vi "Maui 2.0.GetSubpanels.vi"(6 "timeout in ms (-1)":i32, 8 "error in (no error)":errorcluster, 11 "Maui 2.0":refnum<class "Maui 2.0.lvclass">) -> (0 "error out":errorcluster, 2 "Subpanels":refnum<class "SMO.lvclass">[](array[class]), 3 "Maui 2.0 out":refnum<class "Maui 2.0.lvclass">)   [LabVIEW 2020, in "Maui 2.0.lvclass"]
doc: "---------------------------------------------------------------\nJKI State Machine Objects™\nhttp://jki.net/state-machine-objects/\nCopyright (C) 2005-2015, JKI <info@jki.net>\nALL RIGHTS RESERVEDJKI State Machine Objects (SMO) 1.0.0.4\nJKI - JKI\nCopyright (c) 2015, JKI"
uses:
  Maui 2.0.lvclass
  C:/Program Files (x86)/National Instruments/LabVIEW 2020/vi.lib/JKI/JKI SMO/SMO/SMO.lvclass
  <vilib>/JKI/JKI SMO/SMO/SMO.lvclass
  Maui 2.0.lvclass/Maui 2.0.ctl
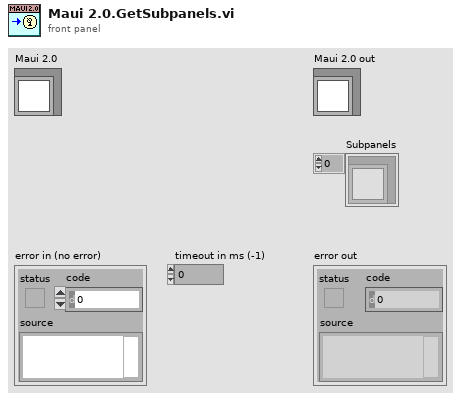
[diagram p1: front panel]
types:
  T1 = typedef "SMO.lvclass/SMOState --Enum.ctl" = enum16{"unknown", "Created", "Started", "Stopped"}
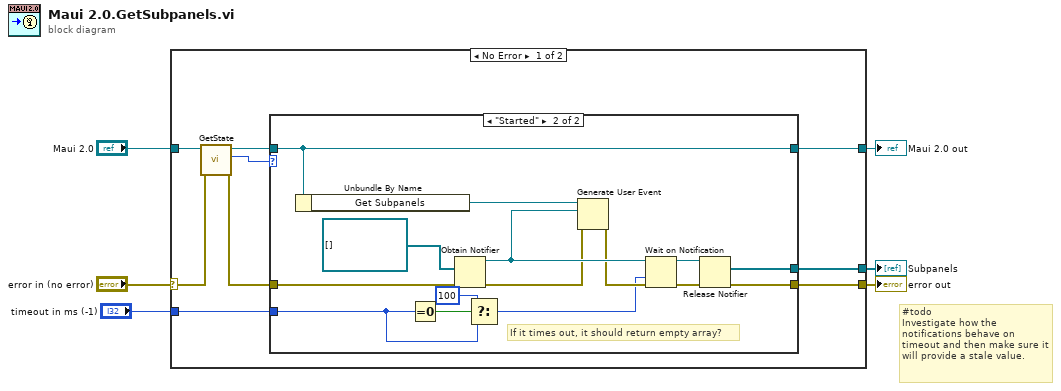
[diagram p0: block diagram]
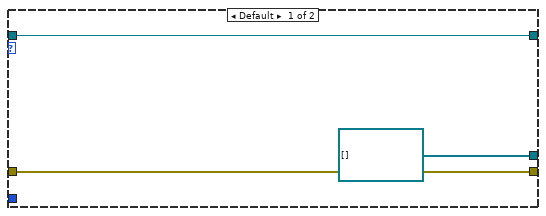
[diagram p2: hidden frame]
diagram:
  # "#todo\nInvestigate how the notifications behave on timeout and then make sure it will provide a stale value."
  n1 = case shown="No Error" "error in (no error)" {
    selector: "error in (no error)" -> [w14 w35]
    tunnel: [w15 w35] -> w6
    tunnel: [w12 w34] -> w4
    tunnel: "Maui 2.0" -> [w10 w34]
    tunnel: [w8 _] -> w1
    tunnel: "timeout in ms (-1)" -> [w7 _]
    frame No Error {
      n2 = call <vilib>:"GetState.vi"("error in (no error)"=w14, "SMO"=w10) -> ("error out"=w13:errorcluster, "SMO State"=w9:T1, "SMO out"=w11:refnum<class "Maui 2.0.lvclass">)  [unwired: 7 in]
      n3 = case shown="\"Started\"" w9 {
        tunnel: [w18 w32] -> w15
        tunnel: w11 -> [w17 w30]
        tunnel: w13 -> [w18 w33]
        tunnel: [w17 w30] -> w12
        tunnel: [refnum<class "SMO.lvclass">[] [] ("Subpanels") w27] -> w8
        tunnel: w7 -> [_ w20]
        frame Default {
        }
        frame "Started" {
          # "If it times out, it should return empty array?"
          n4 = Unbundle By Name(w30) -> ("Get Subpanels"=w31:refnum<user-event>)
          n5 = Equal To 0?(x=w20) -> (x = 0?=w22:bool)
          n6 = Obtain Notifier(notification data type=refnum<class "SMO.lvclass">[] [] ("Subpanels"), error in (no error)=w33) -> (notifier out=w29:refnum<notifier>, error out=w26:errorcluster)  [unwired: 2 in, 1 out]
          n7 = Select(t=100, s=w22, f=w20) -> (s? t:f=w21:i32)
          n8 = Generate User Event(user event=w31, event data cluster=w29, error in=w26) -> (error out=w25:errorcluster)  [unwired: 1 in, 1 out]
          n9 = Wait on Notification(notifier=w29, timeout in ms (-1)=w21, error in (no error)=w25) -> (notifier out=w28:refnum<notifier>, error out=w24:errorcluster)  [unwired: 1 in, 2 out]
          n10 = Release Notifier(notifier=w28, error in (no error)=w24) -> (last notification=w27:refnum<class "SMO.lvclass">[], error out=w32:errorcluster)  [unwired: 1 in, 1 out]
        }
      }
    }
    frame Error {
    }
  }
  "error out" <- w6
  "Maui 2.0 out" <- w4
  "Subpanels" <- w1
